vi "Front Panel.vi"() -> ()   [LabVIEW 2025]
doc: "Author: Scott Hannahs <sth@magnet.fsu.edu>\n\nThis software is licensed for use under the “MIT License\"\nCopyright (c) 2025 Scott Hannahs, sth@sth@magnet.sthnet.net\n\nPermission is hereby granted, free of charge, to any person obtaining a copy of this software and associated documentation files (the \"Software\"), to deal in the Software without restriction, including without limitation the rights to use, copy, modify, merge, publish, distribute, sublicense, and/or sell copies of the Software, and to permit persons to whom the Software is furnished to do so, subject to the following conditions: The above copyright notice and this permission notice shall be included in all copies or substantial portions of the Software.\n\nTHE SOFTWARE IS PROVIDED \"AS IS\", WITHOUT WARRANTY OF ANY KIND, EXPRESS OR IMPLIED, INCLUDING BUT NOT LIMITED TO THE WARRANTIES OF MERCHANTABILITY, FITNESS FOR A PARTICULAR PURPOSE AND NONINFRINGEMENT. IN NO EVENT SHALL THE AUTHORS OR COPYRIGHT HOLDERS BE LIABLE FOR ANY CLAIM, DAMAGES OR OTHER LIABILITY, WHETHER IN AN ACTION OF CONTRACT, TORT OR OTHERWISE, ARISING FROM, OUT OF OR IN CONNECTION WITH THE SOFTWARE OR THE USE OR OTHER DEALINGS IN THE SOFTWARE."
panel:
  in  "NO CHANGES MADE":bool
  in  "CHANGES MADE":bool
  in  "ADJUST SP SR":bool
  in  "SAVE TO FILE":bool
  in  "Path":path
  out "RESET (Inetegral)":dbl min=0.0 max=450.0 step=0.0001 format="%.4f"
  out "RATE (Derivative)":dbl min=0.0 max=450.0 step=0.0001 format="%.4f"
  out "GAIN (Proportional)":dbl min=0.0 max=450.0 step=0.0001 format="%.4f"
  in  "ADJUST PID SETTINGS":bool
  in  "HEATER SETTINGS":bool
  in  "SEND CALIBRATION":bool
  out "TEMPERATURE":dbl(graph)
  out "SAMPLE RATE":dbl=0.292 min=0.0 max=600.0 step=0.0001 format="%.4f"
  out "SET POINT":dbl min=0.0 max=450.0 step=0.0001 format="%.4f"
  out "unit":enum16{"K", "Ohms", "C", "F"}(ring)
  out "Display Temperature":dbl min=0.0 max=450.0 format="%.4f"
  out "MANUAL HEATER SETTING":dbl(slide) scale=0.0..10.0
  out "HEATER Change state bit":bool
  out "Heater DIsplay":bool[](array[boolean])
  # "e"
  # "e"
  # "TEMPERATURE \nREMOTE TEMPERATURE CONTROLLER"
  # "TEMPERATURE \nREMOTE TEMPERATURE CONTROLLER"
  # "SET  POINT"
  # "SET  POINT"
  # "SAMPLE RATE"
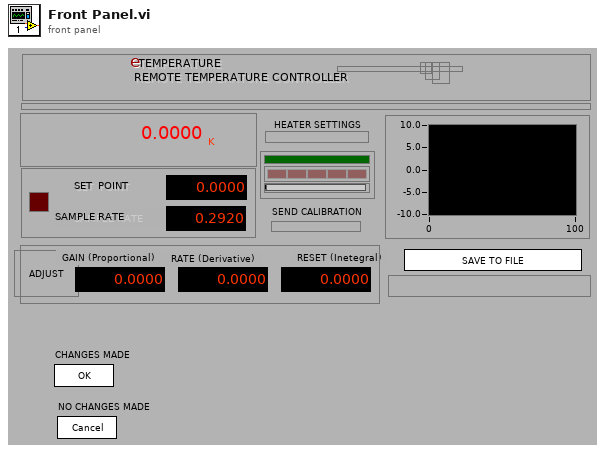
[diagram p1: front panel]
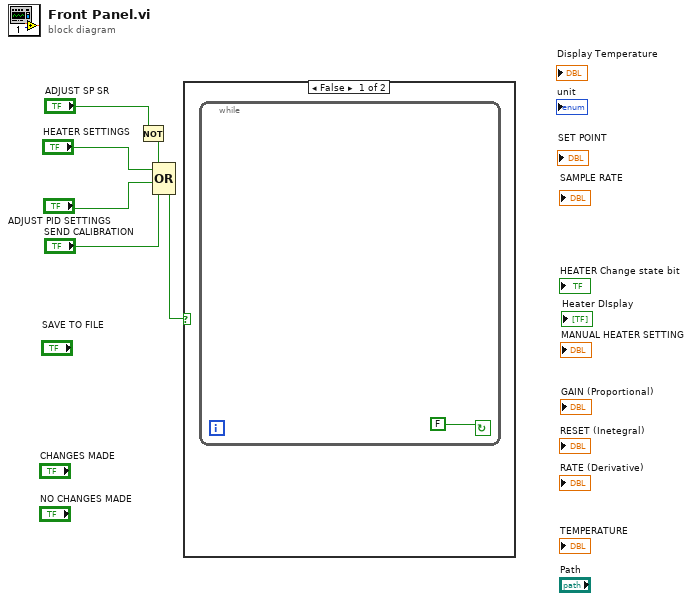
[diagram p0: block diagram]
diagram:
  n1 = Not(x="ADJUST SP SR") -> (.not. x?=w1:bool)
  n2 = Compound Arithmetic op=OR(w1, "HEATER SETTINGS", "ADJUST PID SETTINGS", "SEND CALIBRATION") -> (w2:bool)
  n3 = case shown="False" w2 {
    frame False {
      n4 = while {
        stop <- FALSE continue-if-true
      }
    }
    frame True {
    }
  }
